vi "Set Syringe Valve.vi"(8 "error in (no error)":errorcluster, 9 "Interlock Chain.lvclass":refnum<class "Interlock Chain.lvclass">, 10 "Open? (False)":bool, 11 "Syringe Line in":refnum<class "Syringe Line.lvclass">) -> (0 "error out":errorcluster, 3 "Syringe Line out":refnum<class "Syringe Line.lvclass">)   [LabVIEW 2015, in "cRIO-Carbondioxide.lvlib" / "CO2-Actor.lvlib" / "Syringe Line.lvclass"]
uses:
  Syringe Line.lvclass
  Interlocks/Interlock Chain/Interlock Chain.lvclass
  <vilib>/ActorFramework/Actor/Actor.lvclass/Actor.ctl
  <vilib>/ActorFramework/Message Enqueuer/Message Enqueuer.lvclass/Message Enqueuer.ctl
  Syringe Line.lvclass/Syringe Line.ctl
  Valve Messages/Write Bit Field Msg/Write Bit Field Msg.lvclass/Write Bit Field Msg.ctl
  <vilib>/ActorFramework/Actor/Read Self Enqueuer.vi
  <vilib>/ActorFramework/Message Enqueuer/Enqueue.vi
  <vilib>/ActorFramework/Message Enqueuer/Init from Existing Queue.vi
  <vilib>/ActorFramework/Message Priority Queue/Priority Enqueue.vi
  <vilib>/ActorFramework/Actor/Actor.lvclass
  <vilib>/ActorFramework/Message Enqueuer/Message Enqueuer.lvclass
  Valve Messages/Write Bit Field Msg/Write Bit Field Msg.lvclass
  CO2 Actor/CO2 Actor.lvclass
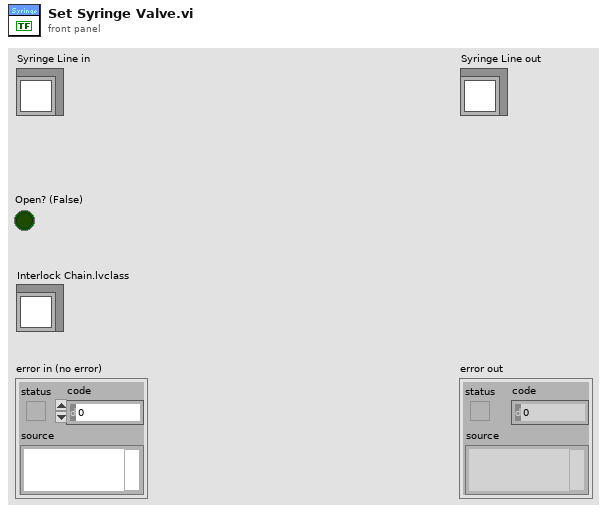
[diagram p1: front panel]
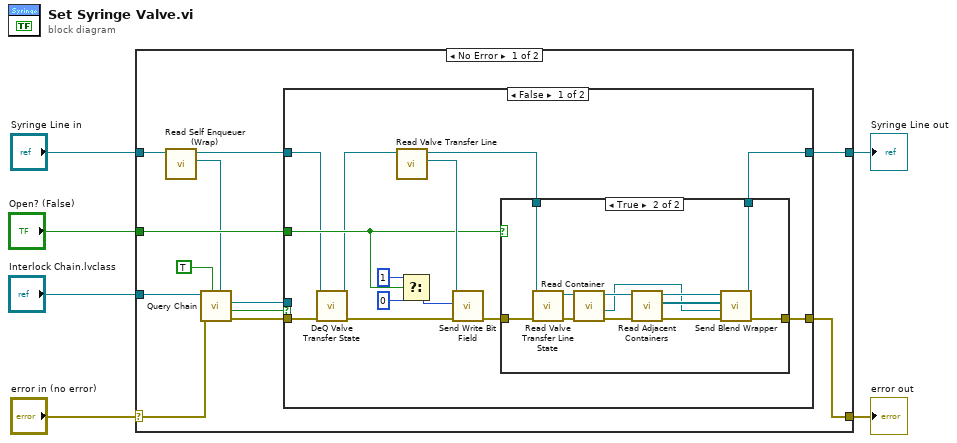
[diagram p0: block diagram]
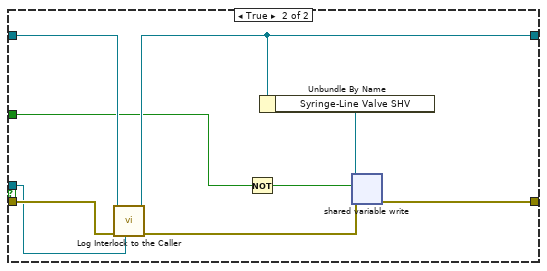
[diagram p3: hidden frame]
diagram:
  n1 = case shown="No Error" "error in (no error)" {
    selector: "error in (no error)" -> [w13 w56]
    tunnel: [w12 w56] -> w5
    tunnel: [w14 w55] -> w3
    tunnel: "Syringe Line in" -> [w9 w55]
    tunnel: "Interlock Chain.lvclass" -> [w18 _]
    tunnel: "Open? (False)" -> [w11 _]
    frame No Error {
      n2 = call "Read Self Enqueuer (Wrap).vi"("CO2 Actor in"=w9) -> ("Actor Framework:Message Enqueuer"=w7:refnum<class "Message Enqueuer.lvclass">, "CO2 Actor out"=w8:refnum<class "Syringe Line.lvclass">)  [unwired: 9 in]
      n3 = call "Query Chain.vi"("Caller Enqueuer"=w7, "Close Connections (F)"=TRUE, "error in (no error)"=w13, "Interlock Chain"=w18) -> ("error out"=w16:errorcluster, "Interlock?"=w17:bool, "Interlock out"=w15:refnum<class "Interlock.lvclass">)  [unwired: 2 in, 3 out]
      n4 = case shown="False" w17 {
        tunnel: w16 -> [w22 w54]
        tunnel: w15 -> [_ w53]
        tunnel: w8 -> [w20 w52]
        tunnel: [w30 w51] -> w14
        tunnel: [w29 w48] -> w12
        tunnel: w11 -> [w26 w47]
        frame False {
          n5 = call "DeQ Valve Transfer State.vi"("error in (no error)"=w22, "Syringe Line in"=w20) -> ("error out"=w21:errorcluster, "Syringe Line out"=w19:refnum<class "Syringe Line.lvclass">)  [unwired: 6 in, 2 out]
          n6 = call "Read Valve Transfer Line.vi"("Syringe Line in"=w19) -> ("Actor Framework:Message Enqueuer"=w27:refnum<class "Message Enqueuer.lvclass">, "Syringe Line out"=w31:refnum<class "Syringe Line.lvclass">)  [unwired: 9 in]
          n7 = Select(t=u16 1, s=w26, f=u16 0 ("Bit Field")) -> (s? t:f=w23:u16)
          n8 = call "Send Write Bit Field.vi"("error in (no error)"=w21, "Bit Field"=w23, "Message Enqueuer"=w27) -> ("error out"=w28:errorcluster)  [unwired: 5 in, 3 out]
          n9 = case shown="True" w26 {
            tunnel: w31 -> [w33 w35]
            tunnel: [w33 w39] -> w30
            tunnel: [w32 w38] -> w29
            tunnel: w28 -> [w32 w37]
            frame False {
            }
            frame True {
              n10 = call "Read Valve Transfer Line State.vi"("error in (no error)"=w37, "Syringe Line in"=w35) -> ("error out"=w36:errorcluster, "Syringe Line out"=w34:refnum<class "Syringe Line.lvclass">)  [unwired: 6 in, 2 out]
              n11 = call "Read Container.vi"("error in (no error)"=w36, "Syringe Line in"=w34) -> ("error out"=w42:errorcluster, "Sample"=w40:refnum<class "Sample.lvclass">, "Syringe Line out"=w41:refnum<class "Syringe Line.lvclass">)  [unwired: 6 in, 1 out]
              n12 = call "Read Adjacent Containers.vi"("error in (no error)"=w42, "Syringe Line in"=w41) -> ("error out"=w44:errorcluster, "Adjacent Containers"=w45:refnum<class "Message Enqueuer.lvclass">[], "Syringe Line out"=w43:refnum<class "Syringe Line.lvclass">)  [unwired: 7 in]
              n13 = call-dynamic "Send Blend Wrapper.vi"("error in (no error)"=w44, "Sample to Blend"=w40, "Send to"=w45, "CO2 Actor in"=w43) -> ("error out"=w38:errorcluster, "CO2 Actor out"=w39:refnum<class "Syringe Line.lvclass">)  [unwired: 6 in]
            }
          }
        }
        frame True {
          n14 = call-dynamic "Log Interlock to the Caller.vi"("Interlock in"=w53, "error in (no error)"=w54, "CO2 Actor in"=w52) -> ("error out"=w49:errorcluster, "CO2 Actor out"=w51:refnum<class "Syringe Line.lvclass">)  [unwired: 7 in]
          n15 = Not(x=w47) -> (.not. x?=w46:bool)
          n16 = Unbundle By Name(w51) -> ("Syringe-Line Valve SHV"=w50:refnum<k21>)
          n17 = shared-variable-write(w50, w49, w46) -> (w48:errorcluster)  [unwired: 1 out]
        }
      }
    }
    frame Error {
    }
  }
  "error out" <- w5
  "Syringe Line out" <- w3
